vi "LabVIEW Sample.vi"() -> ()   [LabVIEW 2010]
panel:
  out "error out":errorcluster {"code" format="%.0x"}
  out "GetConnectState":i32
  out "Data":T1(graph)
  in  "Show Data":bool
  in  "BSACtrl.IBSA":refnum<k7>
  in  "Stop Acq":bool
  in  "Start ACQ":bool
  in  "Processor Properties:":i32(listbox)
  in  "Get Properties":bool
  in  "Disconnect":bool
  in  "Property value":string
  in  "Change value":bool
  in  "Connect state":bool
  in  "IP adress":string="10.10.100.100"
  in  "Connect IP":bool
  in  "Property":i32(listbox)
  in  "stop":bool
  # "IP - Adress:"
  # "Property value:"
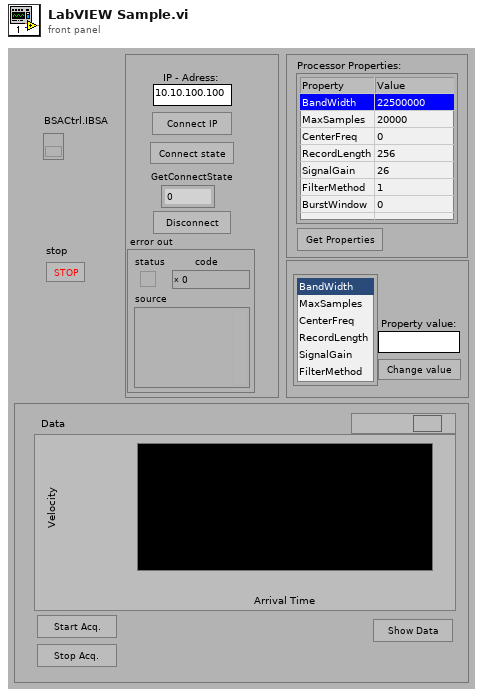
[diagram p1: front panel]
types:
  T1 = cluster{"Array Constant":dbl[], "Array Constant":dbl[]}
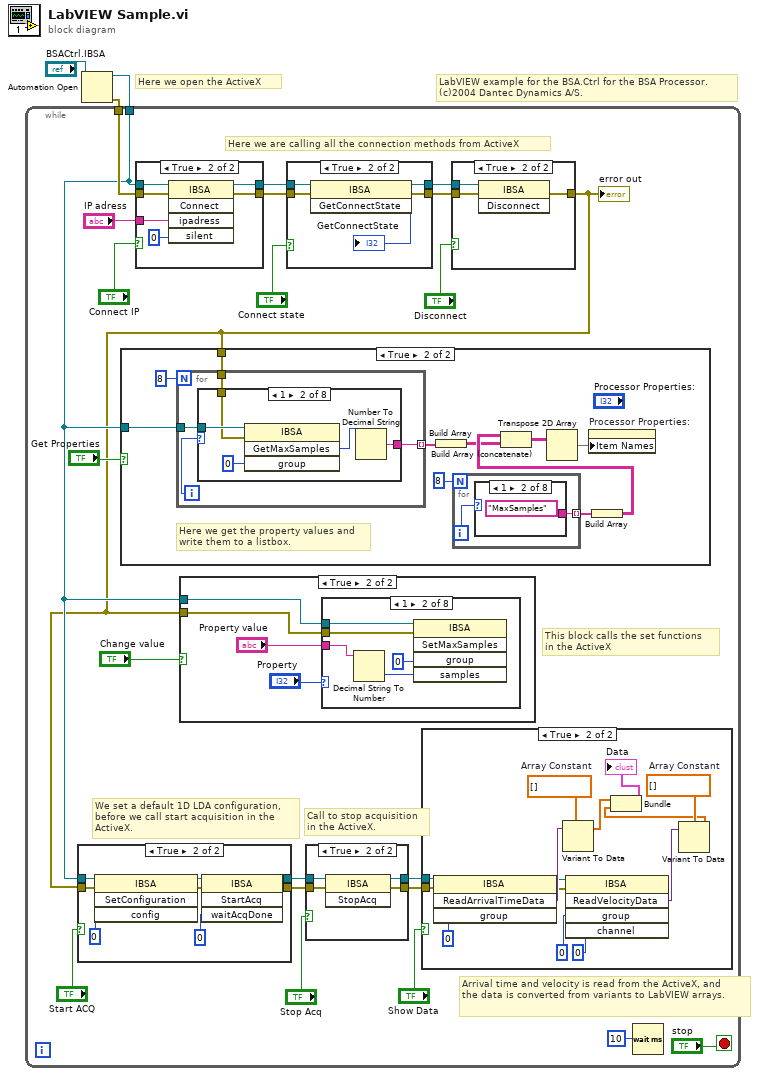
[diagram p0: block diagram]
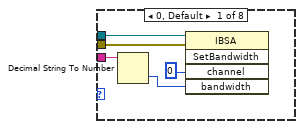
[diagram p6: hidden frame]
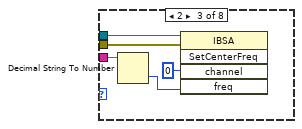
[diagram p7: hidden frame]
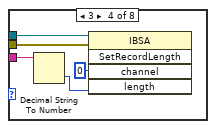
[diagram p8: hidden frame]
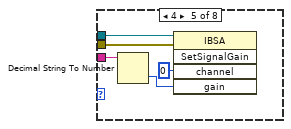
[diagram p9: hidden frame]
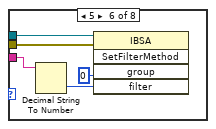
[diagram p10: hidden frame]
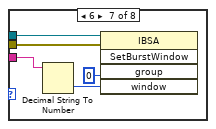
[diagram p11: hidden frame]
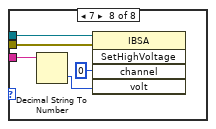
[diagram p12: hidden frame]
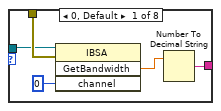
[diagram p14: hidden frame]
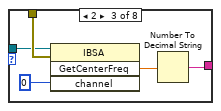
[diagram p15: hidden frame]
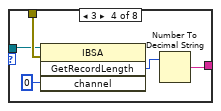
[diagram p16: hidden frame]
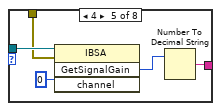
[diagram p17: hidden frame]
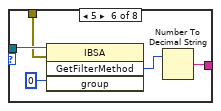
[diagram p18: hidden frame]
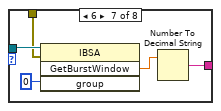
[diagram p19: hidden frame]
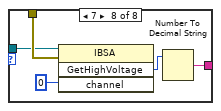
[diagram p20: hidden frame]
diagram:
  # "LabVIEW example for the BSA.Ctrl for the BSA Processor.\n(c)2004 Dantec Dynamics A/S."
  # "Here we open the ActiveX"
  n1 = Automation Open(Automation Refnum="BSACtrl.IBSA") -> (Automation Refnum=w3:refnum<k7>, error out=w1:errorcluster)  [unwired: 3 in]
  n2 = while {
    tunnel: w3 -> [w5]
    tunnel: w1 -> [w15]
    stop <- "stop" stop-if-true
    # "Arrival time and velocity is read from the ActiveX, and \nthe data is converted from variants to LabVIEW arrays."
    # "Call to stop acquisition\nin the ActiveX."
    # "We set a default 1D LDA configuration,\nbefore we call start acquisition in the\nActiveX."
    # "This block calls the set functions\nin the ActiveX"
    # "Here we are calling all the connection methods from ActiveX"
    n3 = case shown="True" "Connect IP" {
      tunnel: [w165 w170] -> w16
      tunnel: [w164 w169] -> w18
      tunnel: "IP adress" -> [_ w168]
      tunnel: w5 -> [w165 w167]
      tunnel: w15 -> [w164 w166]
      frame False {
      }
      frame True {
        n4 = invoke class="IBSA" method="Connect"(reference=w167, error in=w166, "ipadress"=w168, "silent"=0) -> (reference out=w170:refnum<k7>, error out=w169:errorcluster)  [unwired: 1 in, 3 out]
      }
    }
    n5 = case shown="True" "Connect state" {
      tunnel: w16 -> [w173 w178]
      tunnel: [w173 w177] -> w17
      tunnel: w18 -> [w172 w176]
      tunnel: [w172 w175] -> w19
      frame False {
      }
      frame True {
        n6 = invoke class="IBSA" method="GetConnectState"(reference=w178, error in=w176) -> (reference out=w177:refnum<k7>, error out=w175:errorcluster, "GetConnectState"=→"GetConnectState":i32)  [unwired: 1 in]
      }
    }
    n7 = case shown="True" "Disconnect" {
      tunnel: w17 -> [_ w182]
      tunnel: w19 -> [w179 w181]
      tunnel: [w179 w180] -> w4
      frame False {
      }
      frame True {
        n8 = invoke class="IBSA" method="Disconnect"(reference=w182, error in=w181) -> (error out=w180:errorcluster)  [unwired: 1 in, 2 out]
      }
    }
    "error out" <- w4
    n9 = case shown="True" "Start ACQ" {
      tunnel: [w27 w31] -> w9
      tunnel: [w26 w30] -> w10
      tunnel: w5 -> [w27 w29]
      tunnel: w4 -> [w26 w28]
      frame False {
      }
      frame True {
        n10 = invoke class="IBSA" method="SetConfiguration"(reference=w29, error in=w28, "config"=0) -> (reference out=w34:refnum<k7>, error out=w33:errorcluster)  [unwired: 1 in, 2 out]
        n11 = invoke class="IBSA" method="StartAcq"(reference=w34, error in=w33, "waitAcqDone"=0) -> (reference out=w31:refnum<k7>, error out=w30:errorcluster)  [unwired: 1 in, 2 out]
      }
    }
    n12 = case shown="True" "Get Properties" {
      tunnel: w5 -> [_ w101]
      tunnel: w4 -> [_ w100]
      frame False {
      }
      frame True {
        # "Here we get the property values and\nwrite them to a listbox."
        n13 = for {
          N: 8 -> [_]
          tunnel: [w112] -> w103 mode=indexing
          tunnel: w101 -> [w111]
          tunnel: w100 -> [w110]
          i -> [w113]
          n14 = case shown="1" w113 {
            tunnel: [w116 w122 w126 w131 w136 w142 w147 w153] -> w112
            tunnel: w111 -> [w114 w120 w124 w129 w135 w140 w145 w149]
            tunnel: w110 -> [w115 w119 w125 w130 w134 w139 w144 w150]
            frame 0, Default {
              n15 = invoke class="IBSA" method="GetBandwidth"(reference=w114, error in=w115, "channel"=0) -> ("GetBandwidth"=w117:sgl)  [unwired: 1 in, 3 out]
              n16 = Number To Decimal String(number=w117) -> (decimal integer string=w116:string)  [unwired: 1 in]
            }
            frame 1 {
              n17 = invoke class="IBSA" method="GetMaxSamples"(reference=w120, error in=w119, "group"=0) -> ("GetMaxSamples"=w123:i32)  [unwired: 1 in, 3 out]
              n18 = Number To Decimal String(number=w123) -> (decimal integer string=w122:string)  [unwired: 1 in]
            }
            frame 2 {
              n19 = invoke class="IBSA" method="GetCenterFreq"(reference=w124, error in=w125, "channel"=0) -> ("GetCenterFreq"=w127:sgl)  [unwired: 1 in, 3 out]
              n20 = Number To Decimal String(number=w127) -> (decimal integer string=w126:string)  [unwired: 1 in]
            }
            frame 3 {
              n21 = invoke class="IBSA" method="GetRecordLength"(reference=w129, error in=w130, "channel"=0) -> ("GetRecordLength"=w132:i32)  [unwired: 1 in, 3 out]
              n22 = Number To Decimal String(number=w132) -> (decimal integer string=w131:string)  [unwired: 1 in]
            }
            frame 4 {
              n23 = invoke class="IBSA" method="GetSignalGain"(reference=w135, error in=w134, "channel"=0) -> ("GetSignalGain"=w137:i32)  [unwired: 1 in, 3 out]
              n24 = Number To Decimal String(number=w137) -> (decimal integer string=w136:string)  [unwired: 1 in]
            }
            frame 5 {
              n25 = invoke class="IBSA" method="GetFilterMethod"(reference=w140, error in=w139, "group"=0) -> ("GetFilterMethod"=w143:i32)  [unwired: 1 in, 3 out]
              n26 = Number To Decimal String(number=w143) -> (decimal integer string=w142:string)  [unwired: 1 in]
            }
            frame 6 {
              n27 = invoke class="IBSA" method="GetBurstWindow"(reference=w145, error in=w144, "group"=0) -> ("GetBurstWindow"=w148:sgl)  [unwired: 1 in, 3 out]
              n28 = Number To Decimal String(number=w148) -> (decimal integer string=w147:string)  [unwired: 1 in]
            }
            frame 7 {
              n29 = invoke class="IBSA" method="GetHighVoltage"(reference=w149, error in=w150, "channel"=0 ("group")) -> ("GetHighVoltage"=w151:i32)  [unwired: 1 in, 3 out]
              n30 = Number To Decimal String(number=w151) -> (decimal integer string=w153:string)  [unwired: 1 in]
            }
          }
        }
        n31 = Build Array(w103) -> (w107:string[][])
        n32 = for {
          N: 8 -> [_]
          tunnel: [w154] -> w106 mode=indexing
          i -> [w155]
          n33 = case shown="1" w155 {
            tunnel: ["BandWidth" "MaxSamples" "CenterFreq" "RecordLength" "SignalGain" "FilterMethod" "BurstWindow" "HighVoltage"] -> w154
            frame 0, Default {
            }
            frame 1 {
            }
            frame 2 {
            }
            frame 3 {
            }
            frame 4 {
            }
            frame 5 {
            }
            frame 6 {
            }
            frame 7 {
            }
          }
        }
        n34 = Build Array(w106) -> (w108:string[][])
        n35 = Build Array (concatenate)(w108, w107) -> (w104:string[][])
        n36 = Transpose 2D Array(2D array=w104) -> (transposed array=w109:string[][])
        n37 = property on="Processor Properties:" class="MCListbox (strict)"("Item Names"=w109) -> ()  [unwired: 2 in, 2 out]
      }
    }
    n38 = case shown="True" "Change value" {
      tunnel: w4 -> [_ w57]
      tunnel: w5 -> [_ w56]
      frame False {
      }
      frame True {
        n39 = case shown="1" "Property" {
          tunnel: "Property value" -> [w64 w69 w74 w79 w84 w89 w94 w99]
          tunnel: w57 -> [w63 w66 w73 w78 w83 w86 w91 w98]
          tunnel: w56 -> [w62 w65 w72 w77 w82 w85 w90 w97]
          frame 0, Default {
            n40 = Decimal String To Number(string=w64) -> (number=w61:i32)  [unwired: 2 in, 1 out]
            n41 = invoke class="IBSA" method="SetBandwidth"(reference=w62, error in=w63, "channel"=0, "bandwidth"=w61) -> ()  [unwired: 1 in, 5 out]
          }
          frame 1 {
            n42 = Decimal String To Number(string=w69) -> (number=w68:i32)  [unwired: 2 in, 1 out]
            n43 = invoke class="IBSA" method="SetMaxSamples"(reference=w65, error in=w66, "group"=0, "samples"=w68) -> ()  [unwired: 1 in, 5 out]
          }
          frame 2 {
            n44 = Decimal String To Number(string=w74) -> (number=w71:i32)  [unwired: 2 in, 1 out]
            n45 = invoke class="IBSA" method="SetCenterFreq"(reference=w72, error in=w73, "channel"=0, "freq"=w71) -> ()  [unwired: 1 in, 5 out]
          }
          frame 3 {
            n46 = Decimal String To Number(string=w79) -> (number=w76:i32)  [unwired: 2 in, 1 out]
            n47 = invoke class="IBSA" method="SetRecordLength"(reference=w77, error in=w78, "channel"=0, "length"=w76) -> ()  [unwired: 1 in, 5 out]
          }
          frame 4 {
            n48 = Decimal String To Number(string=w84) -> (number=w80:i32)  [unwired: 2 in, 1 out]
            n49 = invoke class="IBSA" method="SetSignalGain"(reference=w82, error in=w83, "channel"=0, "gain"=w80) -> ()  [unwired: 1 in, 5 out]
          }
          frame 5 {
            n50 = Decimal String To Number(string=w89) -> (number=w88:i32)  [unwired: 2 in, 1 out]
            n51 = invoke class="IBSA" method="SetFilterMethod"(reference=w85, error in=w86, "group"=0, "filter"=w88) -> ()  [unwired: 1 in, 5 out]
          }
          frame 6 {
            n52 = Decimal String To Number(string=w94) -> (number=w93:i32)  [unwired: 2 in, 1 out]
            n53 = invoke class="IBSA" method="SetBurstWindow"(reference=w90, error in=w91, "group"=0, "window"=w93) -> ()  [unwired: 1 in, 5 out]
          }
          frame 7 {
            n54 = Decimal String To Number(string=w99) -> (number=w95:i32)  [unwired: 2 in, 1 out]
            n55 = invoke class="IBSA" method="SetHighVoltage"(reference=w97, error in=w98, "channel"=0 ("group"), "volt"=w95) -> ()  [unwired: 1 in, 5 out]
          }
        }
      }
    }
    n56 = case shown="True" "Stop Acq" {
      tunnel: w9 -> [w37 w41]
      tunnel: w10 -> [w36 w40]
      tunnel: [w37 w39] -> w11
      tunnel: [w36 w38] -> w12
      frame False {
      }
      frame True {
        n57 = invoke class="IBSA" method="StopAcq"(reference=w41, error in=w40) -> (reference out=w39:refnum<k7>, error out=w38:errorcluster)  [unwired: 1 in, 1 out]
      }
    }
    n58 = case shown="True" "Show Data" {
      tunnel: w11 -> [_ w43]
      tunnel: w12 -> [_ w42]
      frame False {
      }
      frame True {
        w52 = dbl[] []  # Array Constant
        w54 = dbl[] []  # Array Constant
        n59 = invoke class="IBSA" method="ReadArrivalTimeData"(reference=w43, error in=w42, "group"=0) -> (reference out=w45:refnum<k7>, error out=w44:errorcluster, "ReadArrivalTimeData"=w55:variant)  [unwired: 1 in, 1 out]
        n60 = Variant To Data(Variant=w55, type=w54) -> (data=w49:dbl[])  [unwired: 1 in, 1 out]
        n61 = invoke class="IBSA" method="ReadVelocityData"(reference=w45, error in=w44, "group"=0, "channel"=0 ("ich")) -> ("ReadVelocityData"=w53:variant)  [unwired: 1 in, 4 out]
        n62 = Variant To Data(Variant=w53, type=w52) -> (data=w51:dbl[])  [unwired: 1 in, 1 out]
        n63 = Bundle "Bundle"("Array Constant"=w49, "Array Constant"=w51) -> (→"Data":T1)  [unwired: 1 in]
      }
    }
    n64 = Wait (ms)(milliseconds to wait=u32 10) -> ()  [unwired: 1 out]
  }
